vi "Insight_Discovery_IDN.vi"(8 "error in (no error)":errorcluster, 11 "VISA resource name":refnum<visa-resource-name>) -> (0 "error out":errorcluster, 3 "IDN":string)   [LabVIEW 2014]
panel:
  out "read error":errorcluster
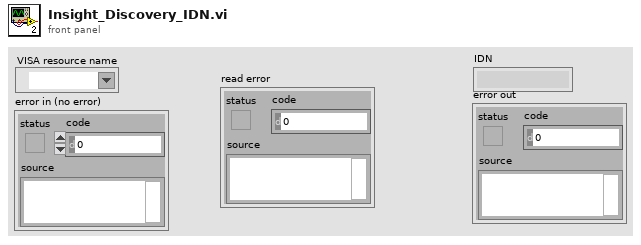
[diagram p1: front panel]
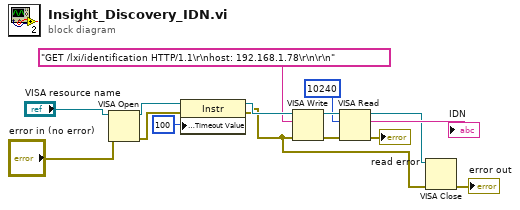
[diagram p0: block diagram]
diagram:
  n1 = VISA Open(error in (no error)="error in (no error)", VISA resource name="VISA resource name") -> (VISA resource name=w11:refnum<visa-resource-name>, error out=w9:errorcluster)  [unwired: 3 in]
  n2 = property class="Instr"(reference=w11, error in=w9, "General Settings:Timeout Value"=u32 100) -> (reference out=w10:refnum<visa-resource-name>, error out=w8:errorcluster)
  n3 = VISA Write(VISA resource name=w10, write buffer="GET /lxi/identification HTTP/1.1\r\nhost: 192.168.1.78\r\n\r\n", error in (no error)=w8) -> (VISA resource name out=w15:refnum<visa-resource-name>, error out=w14:errorcluster)  [unwired: 1 out]
  n4 = VISA Read(VISA resource name=w15, byte count=u32 10240, error in (no error)=w14) -> (VISA resource name out=w4:refnum<visa-resource-name>, read buffer=→"IDN":string, error out=→"read error":errorcluster)  [unwired: 1 out]
  n5 = VISA Close(VISA resource name=w4, error in (no error)=w8) -> (error out=→"error out":errorcluster)
